vi "BK Precision 983X Series Timed Output.vi"() -> ()   [LabVIEW 2015]
doc: "This example configure a timed output."
uses:
  <instrlib>/BK Precision 983X Series/BK Precision 983X Series.lvlib
panel:
  in  "Frequency (50 Hz)":dbl=50.0 min=43.0 max=1200.0 format="%.3g"
  in  "DC Voltage Level (0.0 V)":dbl format="%.3g"
  in  "AC Voltage Level (0.0 V)":dbl format="%.3g"
  in  "Timer Seconds (0)":dbl=2.0 min=0.0 max=59.0 step=1.0 format="%#.1f"
  in  "Timer Minutes (0)":dbl=2.0 min=0.0 max=59.0 step=1.0 format="%#.1f"
  in  "Timer Hour (0)":dbl=2.0 min=0.0 max=999.0 step=1.0 format="%#.1f"
  in  "VISA resource name":refnum<visa-resource-name>
  # "(c) 2017 B&K Precision Corporation.  ALL RIGHTS RESERVED."
  # "hours"
  # "minutes"
  # "seconds"
  # "Hz"
  # "V"
  # "V"
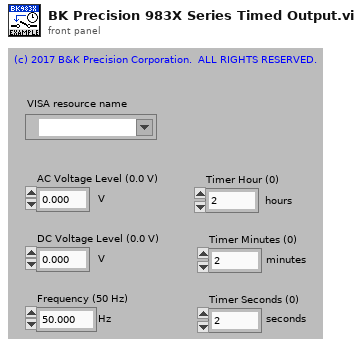
[diagram p1: front panel]
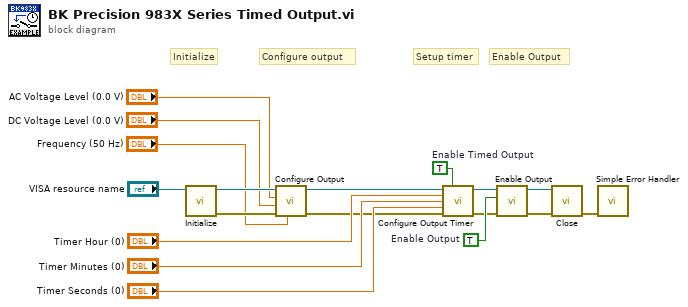
[diagram p0: block diagram]
diagram:
  w5 = TRUE  # Enable Output
  w13 = TRUE  # Enable Timed Output
  # "Enable Output"
  # "Setup timer"
  # "Configure output"
  # "Initialize"
  n1 = call <instrlib>:"Initialize.vi"("VISA resource name"="VISA resource name") -> ("error out"=w11:errorcluster, "VISA resource name out"=w12:refnum<visa-resource-name>)  [unwired: 9 in]
  n2 = call <instrlib>:"Configure Output.vi"("Frequency (50 Hz)"="Frequency (50 Hz)", "error in (no error)"=w11, "DC Voltage Level (0.0 V)"="DC Voltage Level (0.0 V)", "AC Voltage Level (0.0 V)"="AC Voltage Level (0.0 V)", "VISA resource name"=w12) -> ("error out"=w6:errorcluster, "VISA resource name out"=w7:refnum<visa-resource-name>)  [unwired: 5 in]
  n3 = call <instrlib>:"Configure Output Timer.vi"("VISA resource name"=w7, "Enable Timed Output (F: False)"=w13, "Timer Hour (0)"="Timer Hour (0)", "Timer Minutes (0)"="Timer Minutes (0)", "Timer Seconds (0)"="Timer Seconds (0)", "error in (no error)"=w6) -> ("VISA resource name out"=w4:refnum<visa-resource-name>, "error out"=w3:errorcluster)  [unwired: 8 in]
  n4 = call <instrlib>:"Enable Output.vi"("error in (no error)"=w3, "Enable Output (F: False)"=w5, "VISA resource name"=w4) -> ("error out"=w2:errorcluster, "VISA resource name out"=w1:refnum<visa-resource-name>)  [unwired: 7 in]
  n5 = call <instrlib>:"Close.vi"("error in (no error)"=w2, "VISA resource name"=w1) -> ("error out"=w14:errorcluster)  [unwired: 9 in]
  n6 = call <vilib>:"Simple Error Handler.vi"("error in (no error)"=w14) -> ()  [unwired: 4 in, 5 out]
